vi "Barcode_file.vi"(8 "error in":errorcluster, 9 "Read/Write(Read(F))":bool, 10 "Barcode":string, 11 "Barcode_Path":path) -> (0 "error out":errorcluster, 2 "Read_Barcode":string)   [LabVIEW 2024, in "Barcode_Scanner.lvlib"]
uses:
  Barcode_Scanner.lvlib
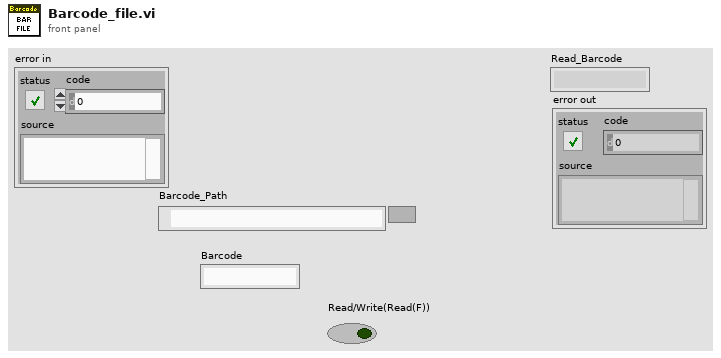
[diagram p1: front panel]
types:
  T1 = enum16{"open", "replace", "create", "open or create", "replace or create", "replace or create with confirmation"}
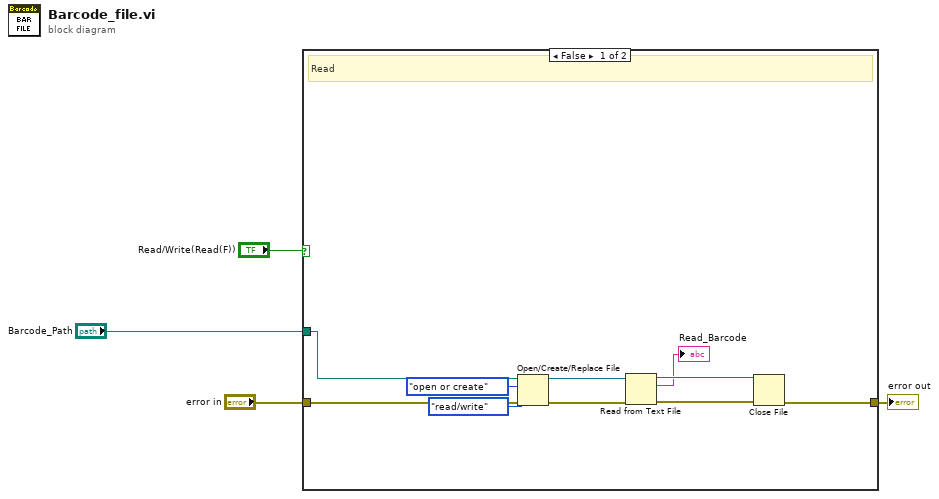
[diagram p0: block diagram]
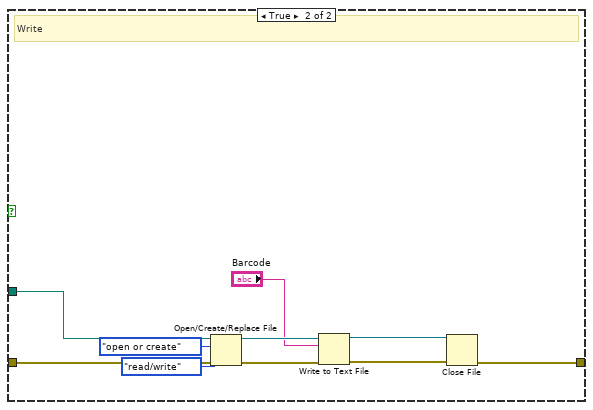
[diagram p2: hidden frame]
diagram:
  n1 = case shown="False" "Read/Write(Read(F))" {
    tunnel: "error in" -> [w8 w24]
    tunnel: "Barcode_Path" -> [w7 w22]
    tunnel: [w5 w15] -> w1
    frame False {
      # "Read"
      n2 = Open/Create/Replace File(file path (use dialog)=w7, error in=w8, operation (0:open)=T1."open or create", access (0:read/write)=enum16{"read/write", "read-only", "write-only"}."read/write") -> (refnum out=w11:refnum<file>, error out=w12:errorcluster)  [unwired: 2 in, 1 out]
      n3 = Read from Text File(file (use dialog)=w11, error in=w12) -> (refnum out=w9:refnum<file>, text=→"Read_Barcode":string, error out=w10:errorcluster)  [unwired: 2 in, 1 out]
      n4 = Close File(refnum=w9, error in=w10) -> (error out=w5:errorcluster)  [unwired: 1 out]
    }
    frame True {
      # "Write"
      n5 = Open/Create/Replace File(file path (use dialog)=w22, error in=w24, operation (0:open)=T1."open or create", access (0:read/write)=enum16{"read/write", "read-only", "write-only"}."read/write") -> (refnum out=w19:refnum<file>, error out=w20:errorcluster)  [unwired: 2 in, 1 out]
      n6 = Write to Text File(file (use dialog)=w19, text="Barcode", error in=w20) -> (refnum out=w16:refnum<file>, error out=w17:errorcluster)  [unwired: 1 in, 1 out]
      n7 = Close File(refnum=w16, error in=w17) -> (error out=w15:errorcluster)  [unwired: 1 out]
    }
  }
  "error out" <- w1
